vi "Switch Status String to Boolean.vi"(1 "String":string caption="Switch") -> (0 "Switch:":bool)   [LabVIEW 2019, in "Instrument.Oxford1820.lvclass"]
uses:
  Instrument.Oxford1820.lvclass
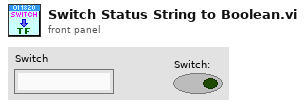
[diagram p1: front panel]
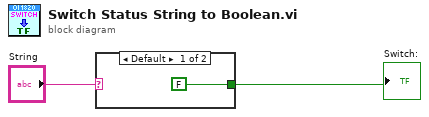
[diagram p0: block diagram]
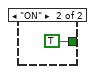
[diagram p2: hidden frame]
diagram:
  n1 = case shown="Default" "String" {
    tunnel: [FALSE TRUE] -> w1
    frame Default {
    }
    frame "ON" {
    }
  }
  "Switch:" <- w1
